vi "Write Data_Write.vi"(8 "error in (no error)":errorcluster, 10 "Data_Write?":bool, 11 "TX Speed in":refnum<class "TX Speed.lvclass">) -> (0 "error out":errorcluster, 3 "TX Speed out":refnum<class "TX Speed.lvclass">)   [LabVIEW 2020, in "TX Speed.lvclass"]
uses:
  TX Speed.lvclass
  TX Speed.lvclass/TX Speed.ctl
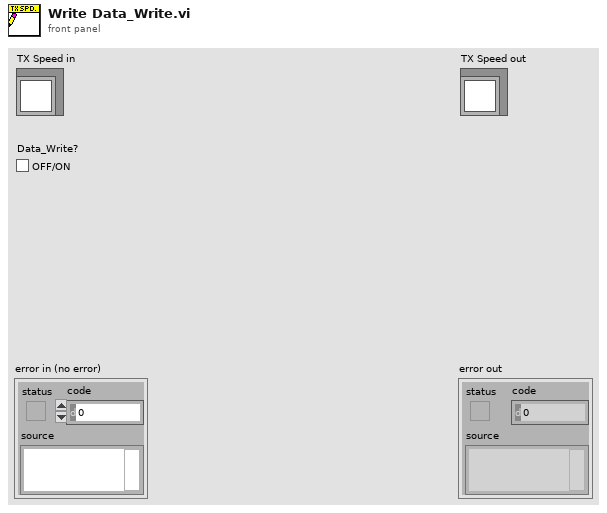
[diagram p1: front panel]
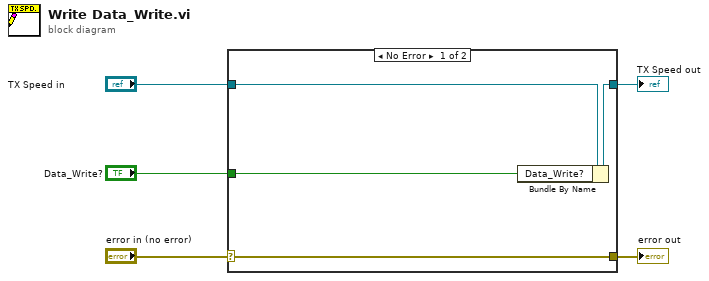
[diagram p0: block diagram]
diagram:
  n1 = case shown="No Error" "error in (no error)" {
    selector: "error in (no error)" -> [w9 w10]
    tunnel: [w9 w10] -> w4
    tunnel: [w7 w11] -> w2
    tunnel: "TX Speed in" -> [w8 w11]
    tunnel: "Data_Write?" -> [w6 _]
    frame No Error {
      n2 = Bundle By Name(cluster=w8, "Data_Write?"=w6) -> (w7:refnum<class "TX Speed.lvclass">)
    }
    frame Error {
    }
  }
  "error out" <- w4
  "TX Speed out" <- w2
